vi "S7_Close_TCP.vi"(8 "error in":errorcluster, 11 "TCP Connection Ref":refnum<k5>) -> (0 "error out":errorcluster)   [LabVIEW 2018, in "S7 TCP.lvlib"]
uses:
  S7 TCP.lvlib
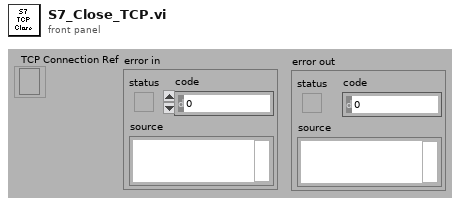
[diagram p1: front panel]
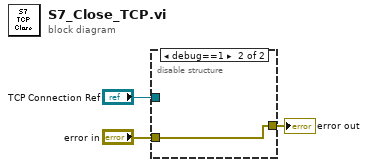
[diagram p0: block diagram]
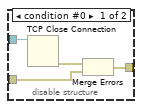
[diagram p2: hidden frame]
diagram:
  n1 = disable-structure shown="debug==1" {
    disable-tunnel: [w7 w8] -> w3
    disable-tunnel: "error in" -> [w5 w8]
    disable-tunnel: "TCP Connection Ref" -> [w4 _]
    frame condition #0 {
      n2 = TCP Close Connection(connection ID=w4) -> (error out=w6:errorcluster)  [unwired: 1 in, 2 out]
      n3 = Merge Errors(w6, w5) -> (w7:errorcluster)
    }
    frame condition #1 (active) {
    }
  }
  "error out" <- w3
